vi "AlazarSamplesPerBuffer.vi"(1 "Records Per Buffer":u32, 2 "Samples Per Record":u32, 4 "Channel Mask":u32) -> (0 "Samples Per Buffer":u32)   [LabVIEW 2021]
doc: "Computes the bytes per buffer given the appropriate input."
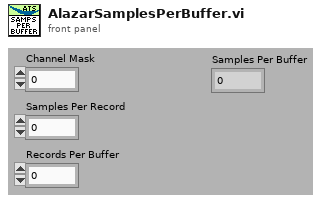
[diagram p1: front panel]
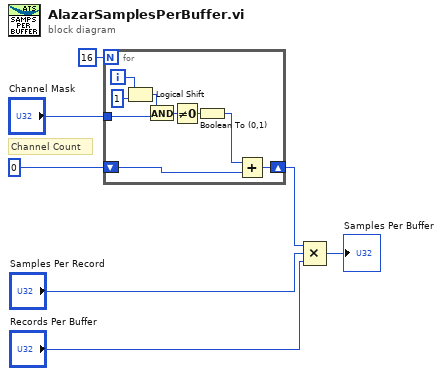
[diagram p0: block diagram]
diagram:
  # "Channel Count"
  n1 = for {
    N: 16 -> [_]
    shift-right: [w15] -> w3
    shift-left: 0 -> [w16]
    tunnel: "Channel Mask" -> [w11]
    i -> [w13]
    n2 = Logical Shift(y=w13, x=u32 1) -> (x << y=w12:u32)
    n3 = And(x=w12, y=w11) -> (x .and. y?=w10:u32)
    n4 = Not Equal To 0?(x=w10) -> (x != 0?=w9:bool)
    n5 = Boolean To (0,1)(Boolean=w9) -> (0, 1=w8:i16)
    n6 = Add(x=w8, y=w16) -> (x+y=w15:i32)
  }
  n7 = Compound Arithmetic op=MULTIPLY(w3, "Samples Per Record", "Records Per Buffer") -> (→"Samples Per Buffer":u32)
